vi "SplineParam_Spline.vi"(11 "inputSPLINE":T5) -> (0 "error out":errorcluster, 3 "outputPOSEwCURVATURE":T1[](array[typedef]) {"POSE"."ROTATION"."SIN" format="%13.4f"; "POSE"."ROTATION"."COS" format="%13.4f"; "POSE"."ROTATION"."VALUE" format="%13.4f"; "POSE"."TRANSLATION"."Y" format="%14.3f"; "POSE"."TRANSLATION"."X" format="%14.3f"})   [LabVIEW 2019, in "Trajectory_Library.lvlib"]
doc: "Parameterizes the spline. This method breaks up the spline into various arcs until their dx, dy, and dtheta are within specific tolerances.\n \nParameters:\n - InputSpline - The spline to parameterize.\n\nReturns:\n - outputPoseWCurvature - A list of poses and curvatures that represents various points on the spline.\n - Error Out - Output error cluster"
uses:
  Trajectory_Library.lvlib
  TypeDef/SPLINE.ctl
  <vilib>/Analysis/Matrix/Datatypes/RealMatrix.ctl
  TypeDef/POSEwCURVATURE.ctl
  TypeDef/POSE2D.ctl
  TypeDef/TRANSLATION2D.ctl
  TypeDef/ROTATION2D.ctl
  <vilib>/Analysis/Matrix/NI_Matrix.lvlib
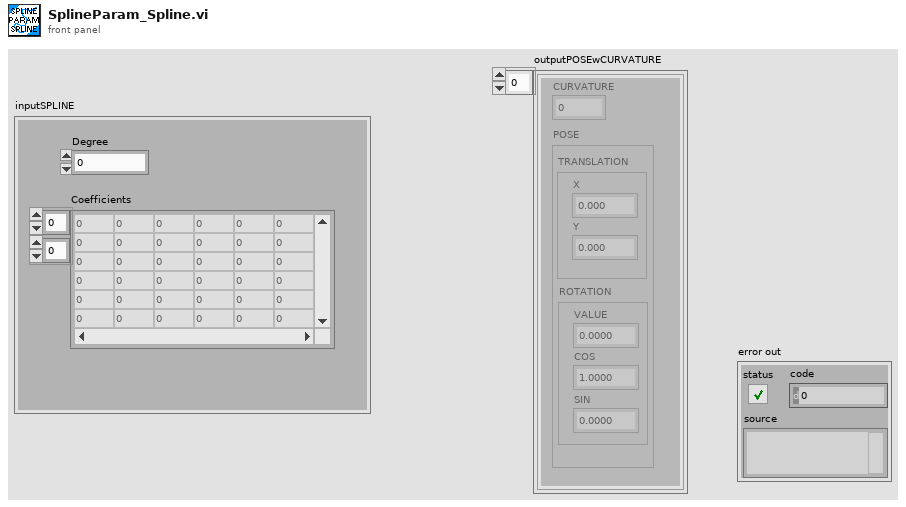
[diagram p1: front panel]
types:
  T1 = typedef "Trajectory_Library.lvlib/POSEwCURVATURE.ctl" = cluster{"CURVATURE":dbl, "POSE":T2}
  T2 = typedef "Trajectory_Library.lvlib/POSE2D.ctl" = cluster{"TRANSLATION":T3, "ROTATION":T4}
  T3 = typedef "Trajectory_Library.lvlib/TRANSLATION2D.ctl" = cluster{"X":dbl, "Y":dbl}
  T4 = typedef "Trajectory_Library.lvlib/ROTATION2D.ctl" = cluster{"VALUE":dbl, "COS":dbl, "SIN":dbl}
  T5 = typedef "Trajectory_Library.lvlib/SPLINE.ctl" = cluster{"Degree":i32, "Coefficients":T6}
  T6 = typedef "NI_Matrix.lvlib/RealMatrix.ctl" = dbl[][]
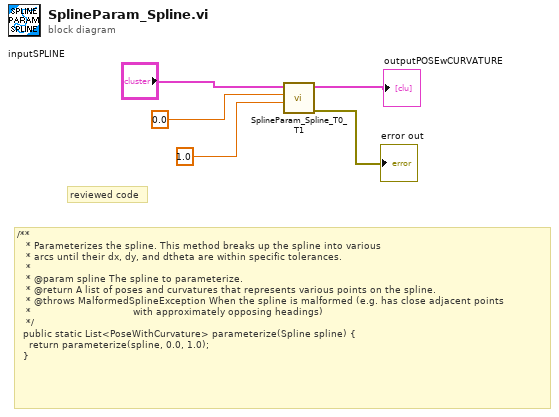
[diagram p0: block diagram]
diagram:
  # "reviewed code"
  # "/**\n   * Parameterizes the spline. This method breaks up the spline into various\n   * arcs until their dx, dy, and dtheta are within specific tolerances.\n   *\n   * @param spline The spline to parameterize.\n   * @return A list of poses and curvatures that represents various points on the spline.\n   * @throws MalformedSplineException When the spline is malformed (e.g. has close adjacent points\n   *                                  with approximately opposing headings)\n   */\n  public static List<PoseWithCurvature> parameterize(Spline spline) {\n    return parameterize(spline, 0.0, 1.0);\n  }"
  n1 = call "SplineParam_Spline_T0_T1.vi"("T1"=1.0, "T0"=0.0, "inputSPLINE"="inputSPLINE") -> ("error out"=→"error out":errorcluster, "outputPOSEwCURVATURE"=→"outputPOSEwCURVATURE":T1[])  [unwired: 7 in]
